vi "DiffKinematics_New.vi"(11 "TrackWidth_Meters":dbl format="%20.4f") -> (3 "DIFF_DRIVE_KINEMATICS":T1 {"TrackWidth_Meters" format="%20.4f"})   [LabVIEW 2019, in "Trajectory_Library.lvlib"]
doc: "Constructs a differential drive kinematics data structure.\n\nHelper class that converts a chassis velocity (dx and dtheta components) to left and right wheel velocities for a differential drive.\n\nInverse kinematics converts a desired chassis speed into left and right velocity components whereas forward kinematics converts left and right component velocities into a linear and angular chassis speed.\n\nParameters: \n - TrackWidthMeters - The track width of the drivetrain. Theoretically, this is the distance between the left wheels and right wheels. However, the empirical value may be larger than the physical measured value due to scrubbing effects.\n\nReturns:\n - Diff Drive Kinematics -- Data structure for Differential Drive Kinematics"
uses:
  Trajectory_Library.lvlib
  TypeDef/DIFF_DRIVE_KINEMATICS.ctl
  <vilib>/Rock Robotics/SystemInterfaces/NetworkCommunication/NetComm_UsageReport_ResourceType.ctl
  Globals/Util_LibraryGlobals.vi
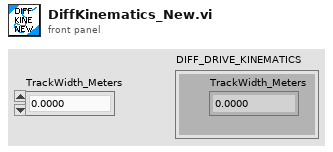
[diagram p1: front panel]
types:
  T1 = typedef "Trajectory_Library.lvlib/DIFF_DRIVE_KINEMATICS.ctl" = cluster{"TrackWidth_Meters":dbl}
  T2 = typedef "NetComm_UsageReport_ResourceType.ctl" = enum8{"Controller", "Module", "Language", "CANPlugin", "Accelerometer", "ADXL345", "AnalogChannel", "AnalogTrigger", "AnalogTriggerOutput", "CANJaguar", "Compressor", "Counter", "Dashboard", "DigitalInput", "DigitalOutput", "DriverStationCIO", "DriverStationEIO", "DriverStationLCD", "Encoder", "GearTooth", "Gyro", "I2C", "Framework", "Jaguar", "Joystick", "Kinect", "KinectStick", "PIDController", "Preferences", "PWM", "Relay", "RobotDrive", "SerialPort", "Servo", "Solenoid", "SPI", "Task", "Ultrasonic", "Victor", "Button", "Command", "AxisCamera", "PCVideoServer", "SmartDashboard", "Talon", "HiTechnicColorSensor", "HiTechnicAccel", "HiTechnicCompass", "SRF08", "AnalogOutput", "Victor SP", "Talon SRX", "CAN Talon SRX", "ADXL362 Accel", "ADXRS450 Gyro", "Rev SPARK", "Mindsensors SD540", "Digital Filter", "ADIS16448", "PDP", "PCM", "PigeonIMU", "Nidec Brushless", "CTRE CANifier", "CTRE TalonFX", "CTRE Future 1", "CTRE Future 2", "CTRE Future 3", "CTRE Future 4", "CTRE Future 5", "CTRE Future 6", "Linear Filter", "Xbox Controller", "USB Camera", "NavX", "Pixy", "Pixy2", "ScanseSweep", "Shuffleboard", "CAN", "Digilent DMC60", "PWM Victor SPX", "Rev SPARK MAX PWM", "Rev SPARK MAX CAN", "ADIS16470", "PIDController2", "ProfiledPIDController", "Kinematics", "Odometry", "Units", "Trapezoid Profile", "DutyCycle", "Addressable LEDs", "Fusion Venom"}
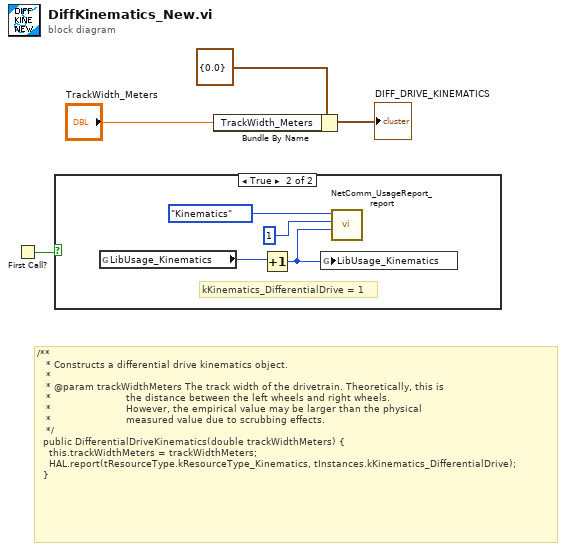
[diagram p0: block diagram]
diagram:
  # "/**\n   * Constructs a differential drive kinematics object.\n   *\n   * @param trackWidthMeters The track width of the drivetrain. Theoretically, this is\n   *                         the distance between the left wheels and right wheels.\n   *                         However, the empirical value may be larger than the physical\n   *                         measured value due to scrubbing effects.\n   */\n  public DifferentialDriveKinematics(double trackWidthMeters) {\n    this.trackWidthMeters = trackWidthMeters;\n    HAL.report(tResourceType.kResourceType_Kinematics, tInstances.kKinematics_DifferentialDrive);\n  }"
  n1 = First Call?() -> (First Call?: T/F=w1:bool)
  n2 = case shown="True" w1 {
    frame False {
    }
    frame True {
      # "kKinematics_DifferentialDrive = 1"
      n3 = global read "Util_LibraryGlobals.vi" "LibUsage_Kinematics"() -> (w7:i32)
      n4 = Increment(x=w7) -> (x+1=w6:i32)
      n5 = global write "Util_LibraryGlobals.vi" "LibUsage_Kinematics"(w6) -> ()
      n6 = call <vilib>:"NetComm_UsageReport_report.vi"("Context"=w6, "Instance Number"=u8 1, "Resource Type"=NetComm_UsageReport_ResourceType."Kinematics") -> ()  [unwired: 9 in]
    }
  }
  n7 = Bundle By Name(cluster=T1 {"TrackWidth_Meters"=0.0} ("DIFF_DRIVE_KINEMATICS"), "TrackWidth_Meters"="TrackWidth_Meters") -> (→"DIFF_DRIVE_KINEMATICS":T1)
